vi "PH_PSDBController.PC set Shottypes.vi"(0 "i ref in":refnum<vi>, 2 "Shottype":i16, 5 "error IO":errorcluster) -> (14 "i ref out":refnum<vi>, 19 "error out":errorcluster)   [LabVIEW 2014, in "PH_PSDBController.lvlib"]
doc: "This sets the Shottype to the GUI and the related DIM service."
uses:
  PH_PSDBController.lvlib
  PH_Basics/PH_PSDBWriter/PH_PSDBWriter.Data Status.ctl
  CSlibraries-extern/DimLVEvent/LVDimInterface/LVDimInterface.lvlib
  CSlibraries-extern/psdb_lv/PSDB.lvlib
  PH_Basics/PH_PSDBWriter/PH_PSDBWriter.lvlib
  PH_Basics/PH_Common/PH_Common.lvlib
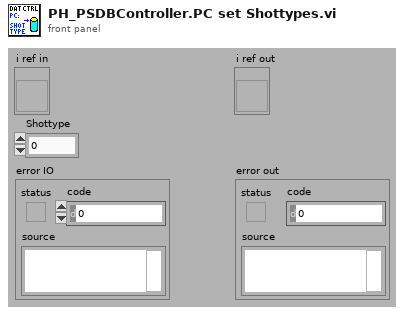
[diagram p1: front panel]
types:
  T1 = typedef "PH_PSDBController.lvlib/PH_PSDBController.i attribute.ctl" = cluster{"GUI Refs":cluster{"Data Status":refnum<vi>, "Current Shot ID":refnum<vi>, "active Subsystems":refnum<vi>, "Experiment Description":refnum<vi>, "Shot Comment":refnum<vi>, "Experiment":refnum<vi>, "Shottype":refnum<vi>, "Sequencer SM State":refnum<vi>, "Instances with Errors":refnum<vi>}, "Service ID Shot ID":i32, "Service ID wanted Subsystem":i32, "Data Status":T2, "Shotinformation":cluster{"Current Experiment ID":i32, "Current Shot Type":i32, "Current Comment":string}, "Data taking?":bool, "Service ID current Shottype":i32, "Service ID current Experiment":i32, "Service ID currentShot Comment":i32, "Service ID possible Shottypes":i32, "Service ID possible Experiments":i32, "possible Experiments":T3[], "possible Shottypes":T3[], "List":cluster{"Info":cluster{"Instance":string, "Data Status":T2}[], "GUI Ref":refnum<vi>, "Classname":string}[], "Subsystems Off?":cluster{"PHELIX_Beamline_fs_YLF_BL_Status":bool, "PHELIX_Beamline_ns_BL_Status":bool, "PHELIX_Beamline_PA_Input_BL_Status":bool, "PHELIX_Beamline_PA_MA_BL_Status":bool, "PHELIX_Beamline_MA_Z6_BL_Status":bool, "PHELIX_Beamline_MA_LB_BL_Status":bool, "PHELIX_Beamline_PA_LL_BL_Status":bool}, "PSDB Credentials":T4}
  T2 = typedef "PH_PSDBWriter.lvlib/PH_PSDBWriter.Data Status.ctl" = i16
  T3 = typedef "PSDB.lvlib/PSDB_Info.ctl" = cluster{"Name":string, "Description":string, "ID":i32}
  T4 = typedef "PH_Common.lvlib/PH_Connection.PSDB Credentials.ctl" = cluster{"PW":string, "ID":string, "DS":string}
  T5 = typedef "NI_Database_API.lvlib/Conn ObjectReference.ctl" = refnum<k1>
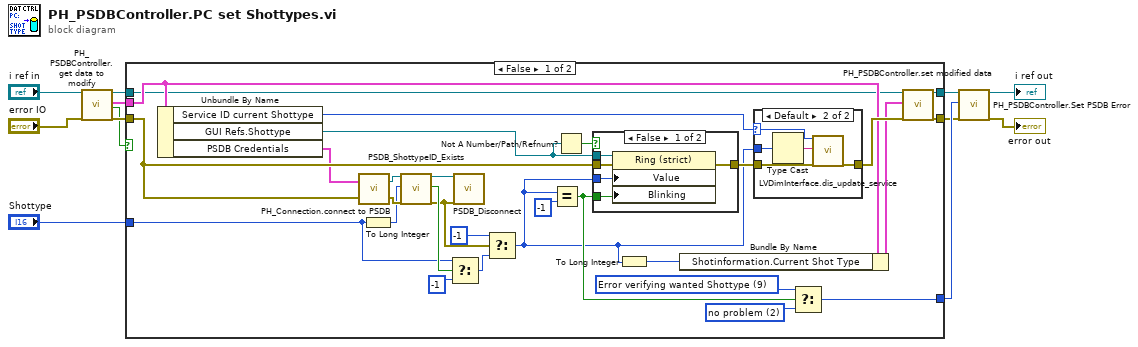
[diagram p0: block diagram]
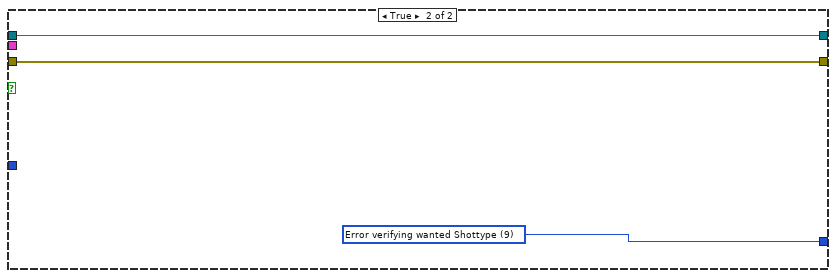
[diagram p4: hidden frame]
diagram:
  n1 = call "PH_PSDBController.get data to modify.vi"("i ref in"="i ref in", "error in (no error)"="error IO") -> ("i ref out"=w4:refnum<vi>, "i attribute"=w10:T1, "timed out"=w1:bool, "error out"=w9:errorcluster)  [unwired: 14 in]
  n2 = case shown="False" w1 {
    tunnel: w10 -> [w16 _]
    tunnel: w9 -> [w15 w55]
    tunnel: [w25 w54] -> w6
    tunnel: "Shottype" -> [w20 _]
    tunnel: w4 -> [w14 w56]
    tunnel: [w24 w56] -> w3
    tunnel: [w23 w55] -> w2
    frame False {
      w26 = T2 2 items=["no info", "no Data collection", "no problem", "Error getting the instance ID", "Error writing Data to data base", "Error concerning the subsystem", "Error getting the Shot ID", "Error getting the Shot Types", "Error getting the Experiments", "Error verifying wanted Shottype", "Error verifying wanted Experiment"] ("Data Status")
      w27 = T2 9 items=["no info", "no Data collection", "no problem", "Error getting the instance ID", "Error writing Data to data base", "Error concerning the subsystem", "Error getting the Shot ID", "Error getting the Shot Types", "Error getting the Experiments", "Error verifying wanted Shottype", "Error verifying wanted Experiment"] ("Data Status")
      n3 = Unbundle By Name(w16) -> ("Service ID current Shottype"=w34:i32, "GUI Refs.Shottype"=w35:refnum<vi>, "PSDB Credentials"=w13:T4)
      n4 = call "PH_Connection.connect to PSDB.vi"("error in"=w15, "PSDB Credentials"=w13) -> ("error out"=w41:errorcluster, "connection reference"=w39:T5)
      n5 = To Long Integer(number=w20) -> (32bit integer=w19:i32)
      n6 = call "PSDB_ShottypeID_Exists.vi"("connection reference"=w39, "shottype_id"=w19, "error in (no error)"=w41) -> ("connection reference out"=w40:T5, "id_exists?"=w38:bool, "error out"=w29:errorcluster)  [unwired: 14 in]
      n7 = Select(t=w20, s=w38, f=i16 -1 ("y")) -> (s? t:f=w30:i16)
      n8 = call "PSDB_Disconnect.vi"("connection reference"=w40, "error in (no error)"=w29) -> ()  [unwired: 17 in, 1 out]
      n9 = Select(t=i16 -1, s=w29, f=w30) -> (s? t:f=w18:i16)
      n10 = Equal?(x=w18, y=i16 -1) -> (x = y?=w28:bool)
      n11 = Not A Number/Path/Refnum?(number/path/refnum=w35) -> (NaN/Path/Refnum?=w37:bool)
      n12 = case shown="False" w37 {
        tunnel: w15 -> [w46 w47]
        tunnel: [w45 w47] -> w33
        tunnel: w35 -> [w44 _]
        tunnel: w18 -> [w42 _]
        tunnel: w28 -> [w43 _]
        frame False {
          n13 = property class="Ring (strict)"(reference=w44, error in=w46, "Value"=w42, "Blinking"=w43) -> (error out=w45:errorcluster)  [unwired: 1 out]
        }
        frame True {
        }
      }
      n14 = To Long Integer(number=w18) -> (32bit integer=w17:i32)
      n15 = Bundle By Name(cluster=w16, "Shotinformation.Current Shot Type"=w17) -> (w21:T1)
      n16 = case shown="Default" w34 {
        selector: w34 -> [_ w51]
        tunnel: [w48 w52] -> w22
        tunnel: w33 -> [w48 w53]
        tunnel: w18 -> [_ w49]
        frame -1 {
        }
        frame Default {
          n17 = Type Cast(x=w49) -> (*(type *) &x=w50:string)  [unwired: 1 in]
          n18 = call "LVDimInterface.dis_update_service.vi"("my_serviceID"=w51, "data"=w50, "error in (no error)"=w53) -> ("error out"=w52:errorcluster)  [unwired: 14 in, 2 out]
        }
      }
      n19 = Select(t=w27, s=w28, f=w26) -> (s? t:f=w25:T2)
      n20 = call "PH_PSDBController.set modified data.vi"("i ref in"=w14, "i attribute"=w21, "error in (no error)"=w22) -> ("i ref out"=w24:refnum<vi>, "error out"=w23:errorcluster)  [unwired: 15 in]
    }
    frame True {
      w54 = T2 9 items=["no info", "no Data collection", "no problem", "Error getting the instance ID", "Error writing Data to data base", "Error concerning the subsystem", "Error getting the Shot ID", "Error getting the Shot Types", "Error getting the Experiments", "Error verifying wanted Shottype", "Error verifying wanted Experiment"] ("Data Status")
    }
  }
  n21 = call "PH_PSDBController.Set PSDB Error.vi"("i ref in"=w3, "Data Status"=w6, "error in"=w2) -> ("i ref out"=→"i ref out":refnum<vi>, "error out"=→"error out":errorcluster)  [unwired: 15 in]
